vi "Test 1050.vi"() -> ()   [LabVIEW 2020]
uses:
  WS1050 1.1/WS1050 1.1.lvclass
  Controls/Change setting mode enum.ctl
  PIC-device/PIC-Device.lvclass
panel:
  out "Last setting 2":bool
  out "Changes 2":cluster{"Name":string, "Value":string}[](array[cluster])
  in  "y":bool
  out "Last setting":bool
  out "Changes":cluster{"Name":string, "Value":string}[][](array[cluster])
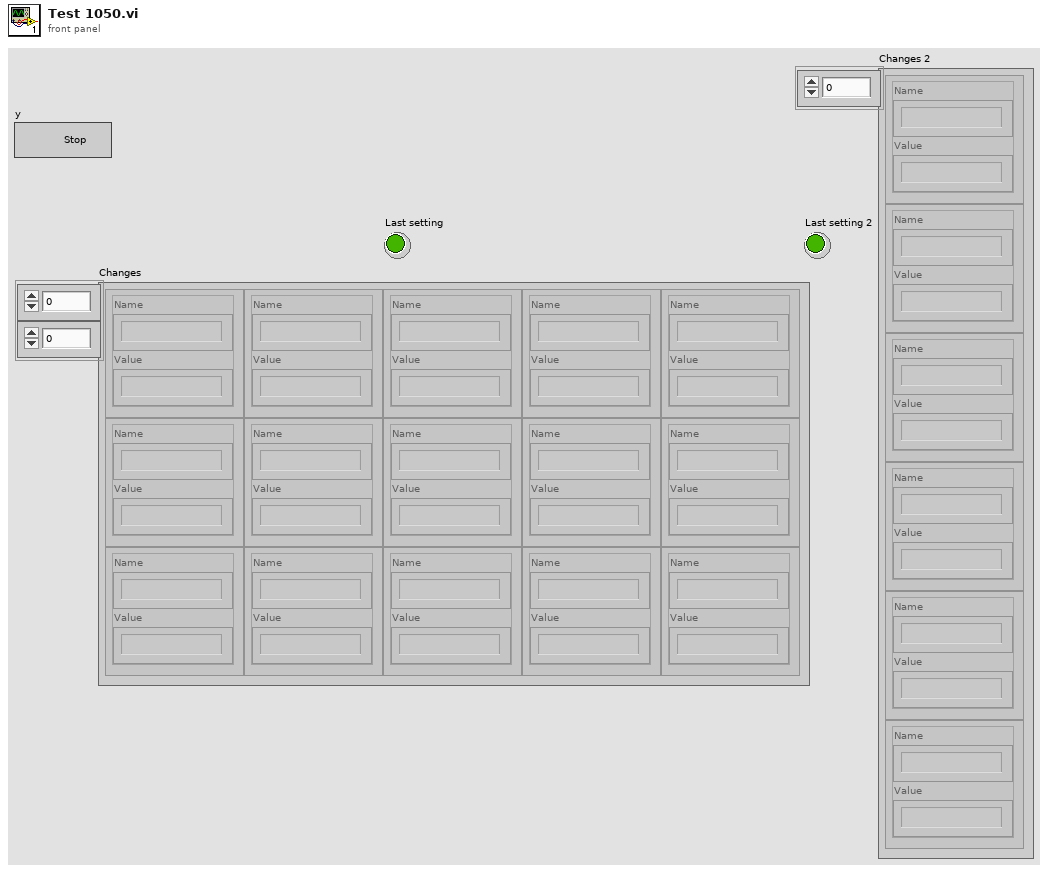
[diagram p1: front panel]
types:
  T1 = typedef "PIC-Device.lvclass/Change setting mode enum.ctl" = enum16{"Init", "Next", "Reset"}
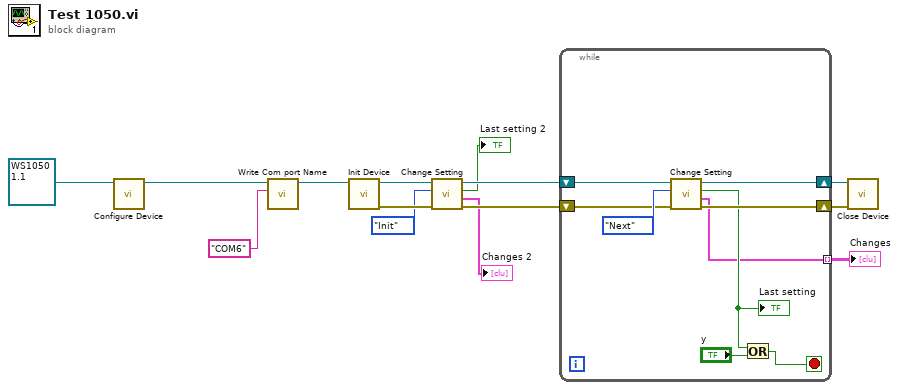
[diagram p0: block diagram]
diagram:
  n1 = call-dynamic "Configure Device.vi"("WS1050 1.1 in"=refnum<class "WS1050 1.1.lvclass"> refnum ("WS1050 1.1.lvclass")) -> ("WS1050 1.1 out"=w12:refnum<class "WS1050 1.1.lvclass">)  [unwired: 9 in, 1 out]
  n2 = call-dynamic "Write Com port Name.vi"("Com port Name"="COM6", "Device in"=w12) -> ("Device out"=w11:refnum<class "WS1050 1.1.lvclass">)  [unwired: 9 in]
  n3 = call-dynamic "Init Device.vi"("Toggle 6 in"=w11) -> ("error out"=w9:errorcluster, "Toggle 6 out"=w10:refnum<class "WS1050 1.1.lvclass">)  [unwired: 9 in]
  n4 = call-dynamic "Change Setting.vi"("error in (no error)"=w9, "Change setting mode"=Change_setting_mode_enum."Init", "Toggle 6 in"=w10) -> ("error out"=w6:errorcluster, "Changes"=→"Changes 2":cluster{"Name":string, "Value":string}[], "Last setting"=→"Last setting 2":bool, "Toggle 6 out"=w7:refnum<class "WS1050 1.1.lvclass">)  [unwired: 5 in]
  n5 = while {
    shift-right: [w19] -> w4
    shift-left: w7 -> [w22]
    shift-right: [w20] -> w5
    shift-left: w6 -> [w21]
    tunnel: [w15] -> w1 mode=indexing
    stop <- w18 stop-if-true
    n6 = call-dynamic "Change Setting.vi"("error in (no error)"=w21, "Change setting mode"=Change_setting_mode_enum."Next", "Toggle 6 in"=w22) -> ("error out"=w20:errorcluster, "Changes"=w15:cluster{"Name":string, "Value":string}[], "Last setting"=w17:bool, "Toggle 6 out"=w19:refnum<class "WS1050 1.1.lvclass">)  [unwired: 5 in]
    "Last setting" <- w17
    n7 = Or(x=w17, y="y") -> (x .or. y?=w18:bool)
  }
  "Changes" <- w1
  n8 = call-dynamic "Close Device.vi"("error in (no error)"=w5, "Device in"=w4) -> ()  [unwired: 8 in, 2 out]
